vi "Tipstrip Mouse Enter (XY Graph).vi"(8 "Error In":errorcluster, 10 "Event Registration Refnum in":refnum<event-registration>, 11 "XYGraph Refnum":refnum<vi>) -> (0 "Error Out":errorcluster, 2 "Event Registration Refnum out":refnum<event-registration>)   [LabVIEW 2021, in "XY Graph Add-Ons.lvlib"]
doc: "Connect the corresponding dynamic event clusters of the Event Structure's \"Mouse Enter\" event for the XYGraph to this subVI"
uses:
  XY Graph/XY Graph Add-Ons.lvlib
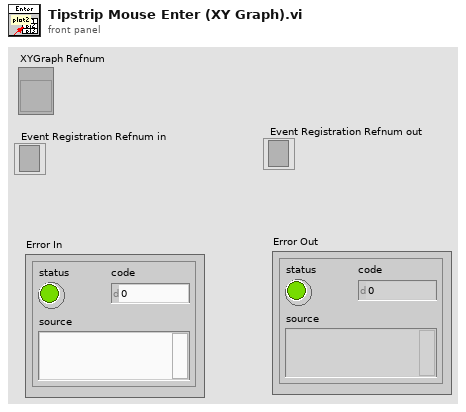
[diagram p1: front panel]
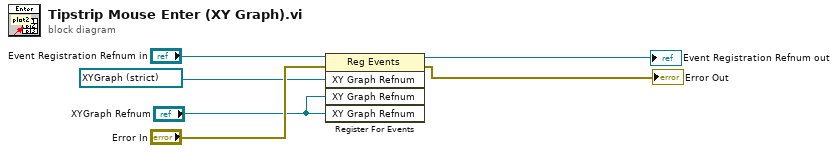
[diagram p0: block diagram]
diagram:
  n1 = register-events(reference="Event Registration Refnum in", error in="Error In", refnum<vi> refnum ("event source"), "XYGraph Refnum", "XYGraph Refnum") -> (reference out=→"Event Registration Refnum out":refnum<event-registration>, error out=→"Error Out":errorcluster)
